vi "Day1.1.vi"() -> ()   [LabVIEW 2023]
panel:
  out "Sum":i32
  out "Array":i32[](array[numeric])
  out "B":i32[](array[numeric])
  out "A":i32[](array[numeric])
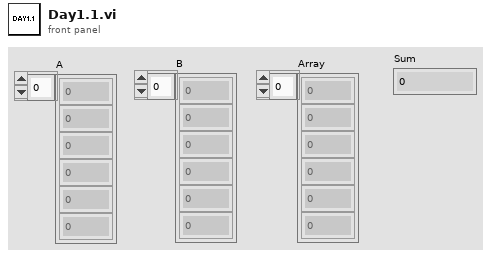
[diagram p1: front panel]
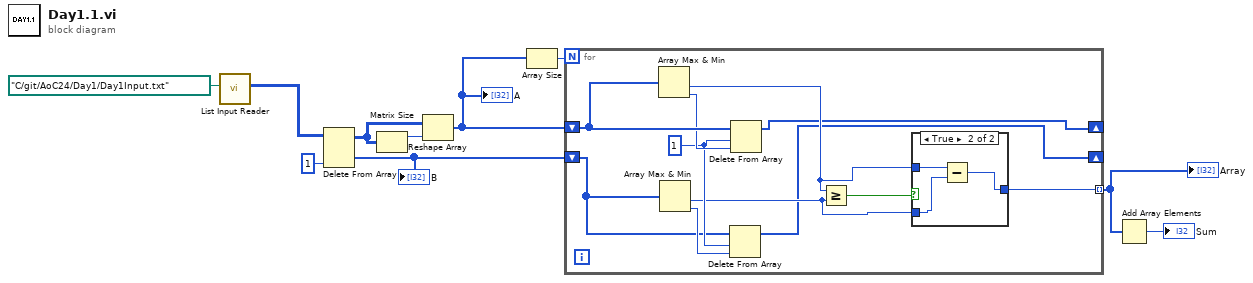
[diagram p0: block diagram]
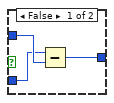
[diagram p2: hidden frame]
diagram:
  n1 = call "List Input Reader.vi"("file path (dialog if empty)"=path "C:/git/AoC24/Day1/Day1Input.txt") -> ("Array"=w9:i32[][])  [unwired: 9 in, 1 out]
  n2 = Delete From Array(array=w9, index (col)=1 ("disabled index (col)")) -> (deleted portion=w5:i32[], array with subset deleted=w7:i32[][])  [unwired: 2 in]
  "B" <- w5
  n3 = Matrix Size(0:w7) -> (1:w6:i32)  [unwired: 1 out]
  n4 = Reshape Array(w7, w6) -> (w3:i32[])
  "A" <- w3
  n5 = Array Size(array=w3) -> (size(s)=w4:i32)
  n6 = for {
    N: w4 -> [_]
    shift-right: [w12] -> _
    shift-left: w3 -> [w21]
    shift-right: [w13] -> _
    shift-left: w5 -> [w14]
    tunnel: [w15] -> w2 mode=indexing
    w19 = 1 ("length")
    n7 = Array Max & Min(array=w21) -> (min value=w17:i32, min index (indices)=w20:i32)  [unwired: 2 out]
    n8 = Array Max & Min(array=w14) -> (min value=w16:i32, min index (indices)=w18:i32)  [unwired: 2 out]
    n9 = Delete From Array(array=w14, length=w19, index=w18) -> (array with subset deleted=w13:i32[])  [unwired: 1 out]
    n10 = Delete From Array(array=w21, length=w19, index=w20) -> (array with subset deleted=w12:i32[])  [unwired: 1 out]
    n11 = Greater Or Equal?(x=w17, y=w16) -> (x >= y?=w11:bool)
    n12 = case shown="True" w11 {
      tunnel: w17 -> [w24 w27]
      tunnel: w16 -> [w23 w26]
      tunnel: [w22 w25] -> w15
      frame False {
        n13 = Subtract(x=w23, y=w24) -> (x-y=w22:i32)
      }
      frame True {
        n14 = Subtract(x=w27, y=w26) -> (x-y=w25:i32)
      }
    }
  }
  "Array" <- w2
  n15 = Add Array Elements(numeric array=w2) -> (sum=→"Sum":i32)
